vi "Run.vi"(8 "error in (no error)":errorcluster caption="entrée d'erreur (pas d'erreur)", 11 "20newsgroups_vectorized.lvclass":refnum<class "20newsgroups_vectorized.lvclass">) -> (0 "error out":errorcluster caption="sortie d'erreur", 2 "Data":T1, 3 "20newsgroups_vectorized.lvclass 2":refnum<class "20newsgroups_vectorized.lvclass">)   [LabVIEW 2020, in "20newsgroups_vectorized.lvclass"]
doc: "Get data : sparse matrix, shape [n_samples, n_features]\n The data matrix to learn."
uses:
  20newsgroups_vectorized.lvclass
  20newsgroups_vectorized.lvclass/20newsgroups_vectorized.ctl
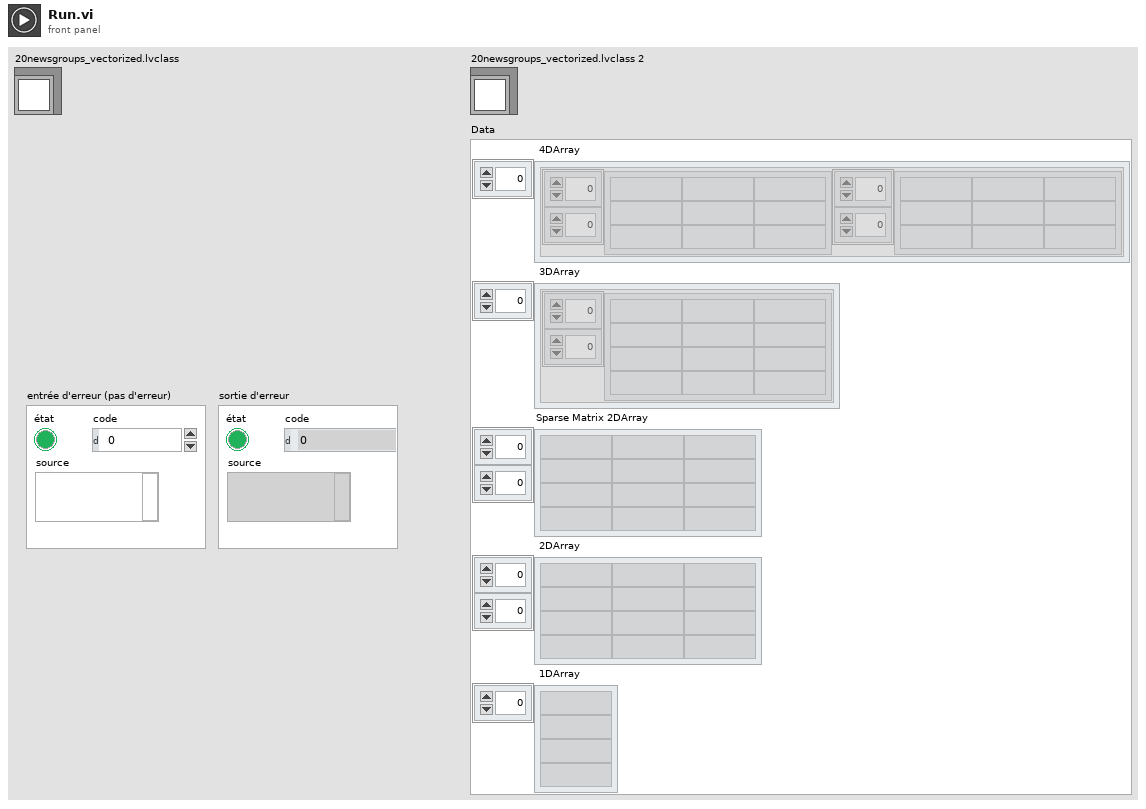
[diagram p1: front panel]
types:
  T1 = cluster{" 4DArray":cluster{"1":string[][], "2":string[][]}[], " 3DArray":cluster{"Tableau":string[][]}[], "Sparse Matrix 2DArray":string[][], " 2DArray":string[][], " 1DArray":string[]}
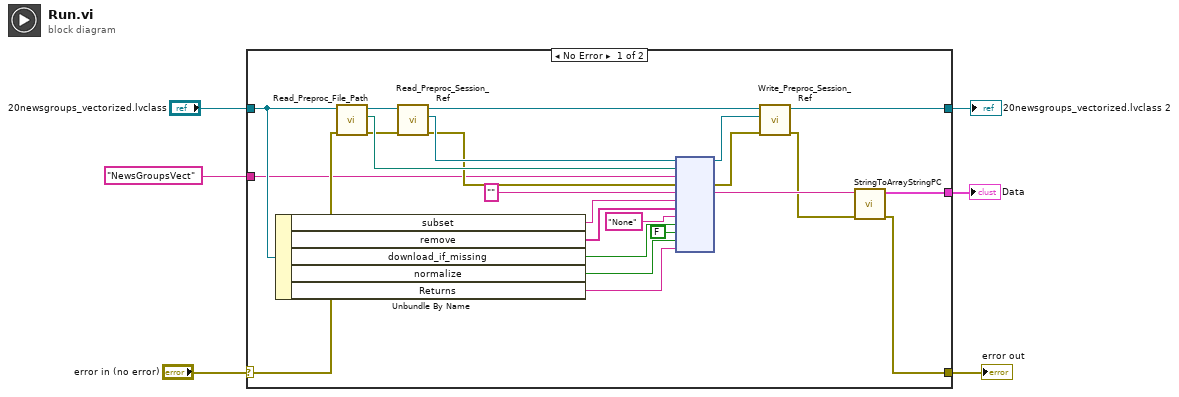
[diagram p0: block diagram]
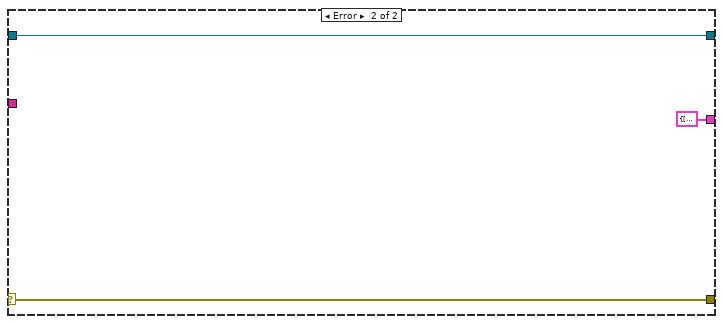
[diagram p2: hidden frame]
diagram:
  n1 = case shown="No Error" "error in (no error)" {
    selector: "error in (no error)" -> [w21 w33]
    tunnel: [w8 w33] -> w5
    tunnel: [w11 w32] -> w1
    tunnel: "20newsgroups_vectorized.lvclass" -> [w20 w32]
    tunnel: "NewsGroupsVect" -> [w19 _]
    tunnel: [w7 T1 {" 4DArray"=[], " 3DArray"=[], "Sparse Matrix 2DArray"=[], " 2DArray"=[], " 1DArray"=[]} ("Data")] -> w4
    frame No Error {
      n2 = Unbundle By Name(w20) -> ("subset"=w18:string, "remove"=w17:string[], "download_if_missing"=w15:bool, "normalize"=w13:bool, "Returns"=w12:string)
      n3 = call-dynamic "Read_Preproc_File_Path.vi"("error in (no error)"=w21, "Python in"=w20) -> ("error out"=w25:errorcluster, "File_Path"=w28:path, "Python out"=w30:refnum<class "20newsgroups_vectorized.lvclass">)  [unwired: 7 in]
      n4 = call-dynamic "Read_Preproc_Session_Ref.vi"("error in (no error)"=w25, "Python in"=w30) -> ("error out"=w26:errorcluster, "Session_ref"=w27:refnum<k35>, "Python out"=w29:refnum<class "20newsgroups_vectorized.lvclass">)  [unwired: 7 in]
      n5 = node(w27, w28, w19, w26, "", w18, w17, "None", w15, FALSE, w13, w12) -> (w22:refnum<k35>, w24:errorcluster, w10:string)  [unwired: 7 in, 2 out]
      n6 = call-dynamic "Write_Preproc_Session_Ref.vi"("error in (no error)"=w24, "Session_ref"=w22, "Python in"=w29) -> ("error out"=w9:errorcluster, "Python out"=w11:refnum<class "20newsgroups_vectorized.lvclass">)  [unwired: 7 in]
      n7 = call "StringToArrayStringPC.vi"("sortie d'erreur"=w9, "Return value"=w10) -> ("sortie d'erreur"=w8:errorcluster, "Data"=w7:T1)  [unwired: 8 in]
    }
    frame Error {
    }
  }
  "error out" <- w5
  "Data" <- w4
  "20newsgroups_vectorized.lvclass 2" <- w1
